vi "查询产品ID-14.vi"(8 "error in (no error)":errorcluster, 11 "芯片编码":string) -> (0 "error out":errorcluster, 2 "产品ID":string, 3 "索引结果":bool)   [LabVIEW 2013]
uses:
  <vilib>/Utility/error.llb/whitespace.ctl
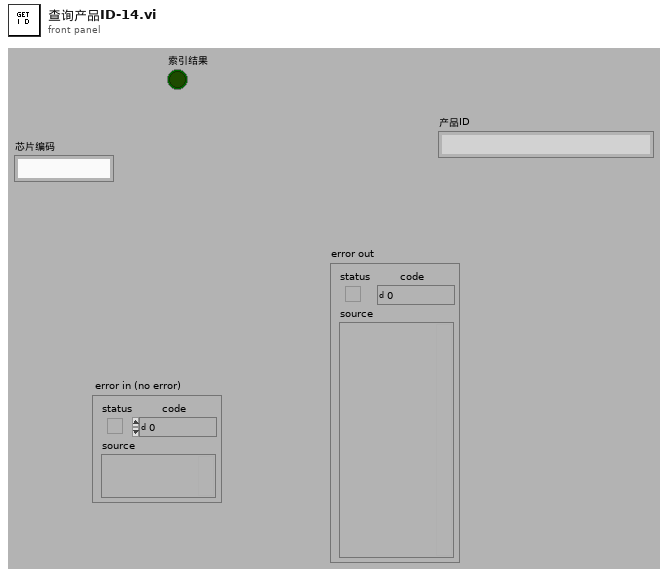
[diagram p1: front panel]
types:
  T1 = typedef "whitespace.ctl" = u16
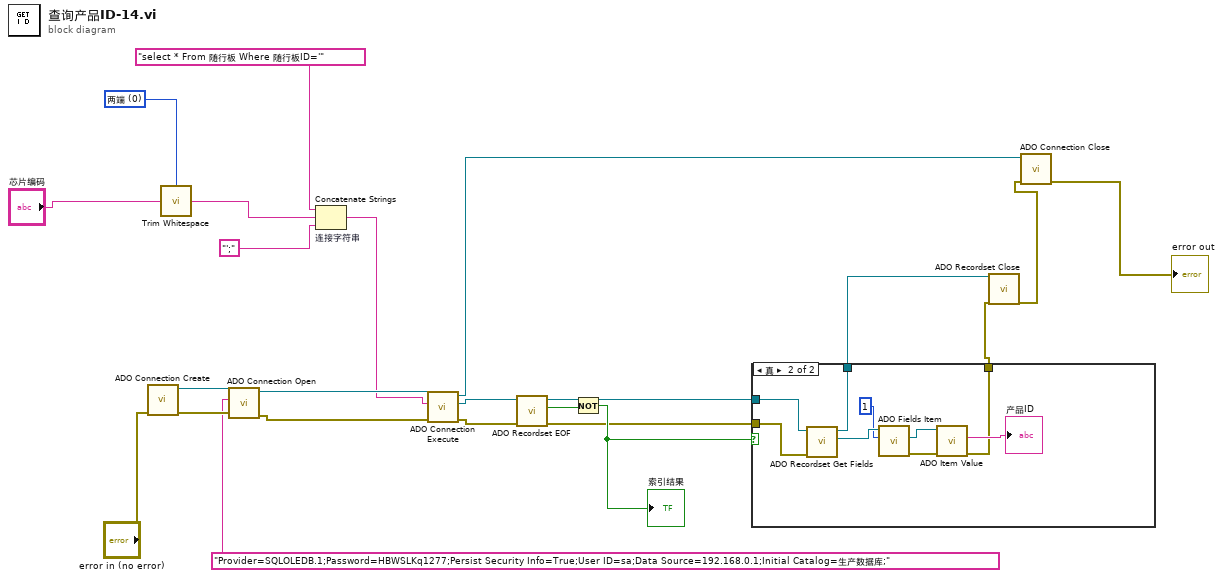
[diagram p0: block diagram]
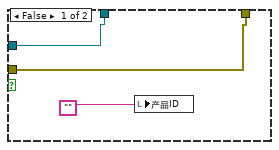
[diagram p2: hidden frame]
diagram:
  w10 = T1 0 items=["两端", "字符串首端", "字符串末端"] ("location (both)")
  n1 = call "ADO Connection Create.vi"("error in (no error)"="error in (no error)") -> ("error out"=w22:errorcluster, "ADODB._Connection Out"=w23:refnum<k7>)  [unwired: 9 out]
  n2 = call <vilib>:"Trim Whitespace.vi"("string"="芯片编码", "location (both)"=w10) -> ("trimmed string"=w11:string)
  n3 = call "ADO Connection Open.vi"("error in (no error)"=w22, "ConnectionString"="Provider=SQLOLEDB.1;Password=HBWSLKq1277;Persist Security Info=True;User ID=sa;Data Source=192.168.0.1;Initial Catalog=生产数据库;" ("字符串 2"), "ADODB._Connection In"=w23) -> ("error out"=w21:errorcluster, "ADODB._Connection Out"=w20:refnum<k7>)  [unwired: 7 out]
  n4 = Concatenate Strings "连接字符串"("select * From 随行板 Where 随行板ID='" ("字符串 2"), w11, "';" ("字符串 2")) -> (w9:string)
  n5 = call "ADO Connection Execute.vi"("error in (no error)"=w21, "CommandText"=w9, "ADODB._Connection In"=w20) -> ("error out"=w17:errorcluster, "RecordSet"=w18:refnum<k7>, "ADODB._Connection Out"=w14:refnum<k7>)  [unwired: 6 out]
  n6 = call "ADO Recordset EOF.vi"("error in (no error)"=w17, "ADODB._Recordset In"=w18) -> ("error out"=w4:errorcluster, "EOF"=w16:bool, "ADODB._Recordset Out"=w5:refnum<k7>)  [unwired: 7 out]
  n7 = Not(x=w16) -> (.not. x?=w6:bool)
  "索引结果" <- w6
  n8 = case shown="真" w6 {
    tunnel: w5 -> [w25 w35]
    tunnel: w4 -> [w26 w34]
    tunnel: [w25 w33] -> w3
    tunnel: [w26 w27] -> w2
    frame False {
      n9 = local write "产品ID"("") -> ()
    }
    frame True {
      n10 = call "ADO Recordset Get Fields.vi"("error in (no error)"=w34, "ADODB._Recordset In"=w35) -> ("Fields Out"=w32:refnum<k7>, "ADODB._Recordset Out"=w33:refnum<k7>)  [unwired: 8 out]
      n11 = call "ADO Fields Item.vi"("Index"=1, "Fields In"=w32) -> ("error out"=w30:errorcluster, "Item Out"=w29:refnum<k7>)  [unwired: 1 in, 7 out]
      n12 = call "ADO Item Value.vi"("error in (no error)"=w30, "Item In"=w29) -> ("error out"=w27:errorcluster, "Value"=→"产品ID":string)  [unwired: 8 out]
    }
  }
  n13 = call "ADO Recordset Close.vi"("ADODB._Recordset In"=w3, "error in (no error)"=w2) -> ("error out"=w15:errorcluster)  [unwired: 17 out]
  n14 = call "ADO Connection Close.vi"("error in (no error)"=w15, "ADODB._Connection In"=w14) -> ("error out"=→"error out":errorcluster)  [unwired: 9 out]
